vi "Std_dilution_SubVI_BM.vi"(6 "COM Port":refnum<visa-resource-name>="COM9", 7 "Pump Parameters":T1={"Speed 1"="100", "Speed 2"="250", "Speed 3"="250", "Speed 4"="250", "UW/Sample"="5", "Sparge"="2", "Std"="4", "Waste"="15", "Air"="14", "Milli-Q"="1", "H2SO4"="6", "NaOH"="3", "Catalyst"="7", "Cell (H+ side)"="8", "Cell (sample side)"="9", "NaCl"="9"}, 9 "step to ml":dbl=1920.0, 10 "Total Vol. (mL)":dbl, 11 "Dilution Vol. (mL)":dbl=10.0) -> ()   [LabVIEW 2021]
panel:
  out "Full Command":string="o4A0V5000o1P14400o4D14400o1P33600o4D9600o2D24000o5P9600o2D9600o6P33600o4D33600"
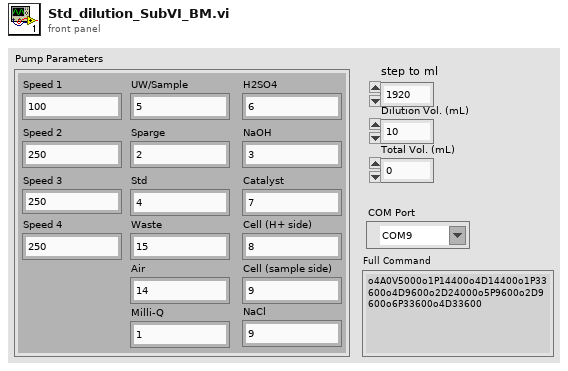
[diagram p1: front panel]
types:
  T1 = cluster{"Speed 1":string, "Speed 2":string, "Speed 3":string, "Speed 4":string, "UW/Sample":string, "Sparge":string, "Std":string, "Waste":string, "Air":string, "Milli-Q":string, "H2SO4":string, "NaOH":string, "Catalyst":string, "Cell (H+ side)":string, "Cell (sample side)":string, "NaCl":string}
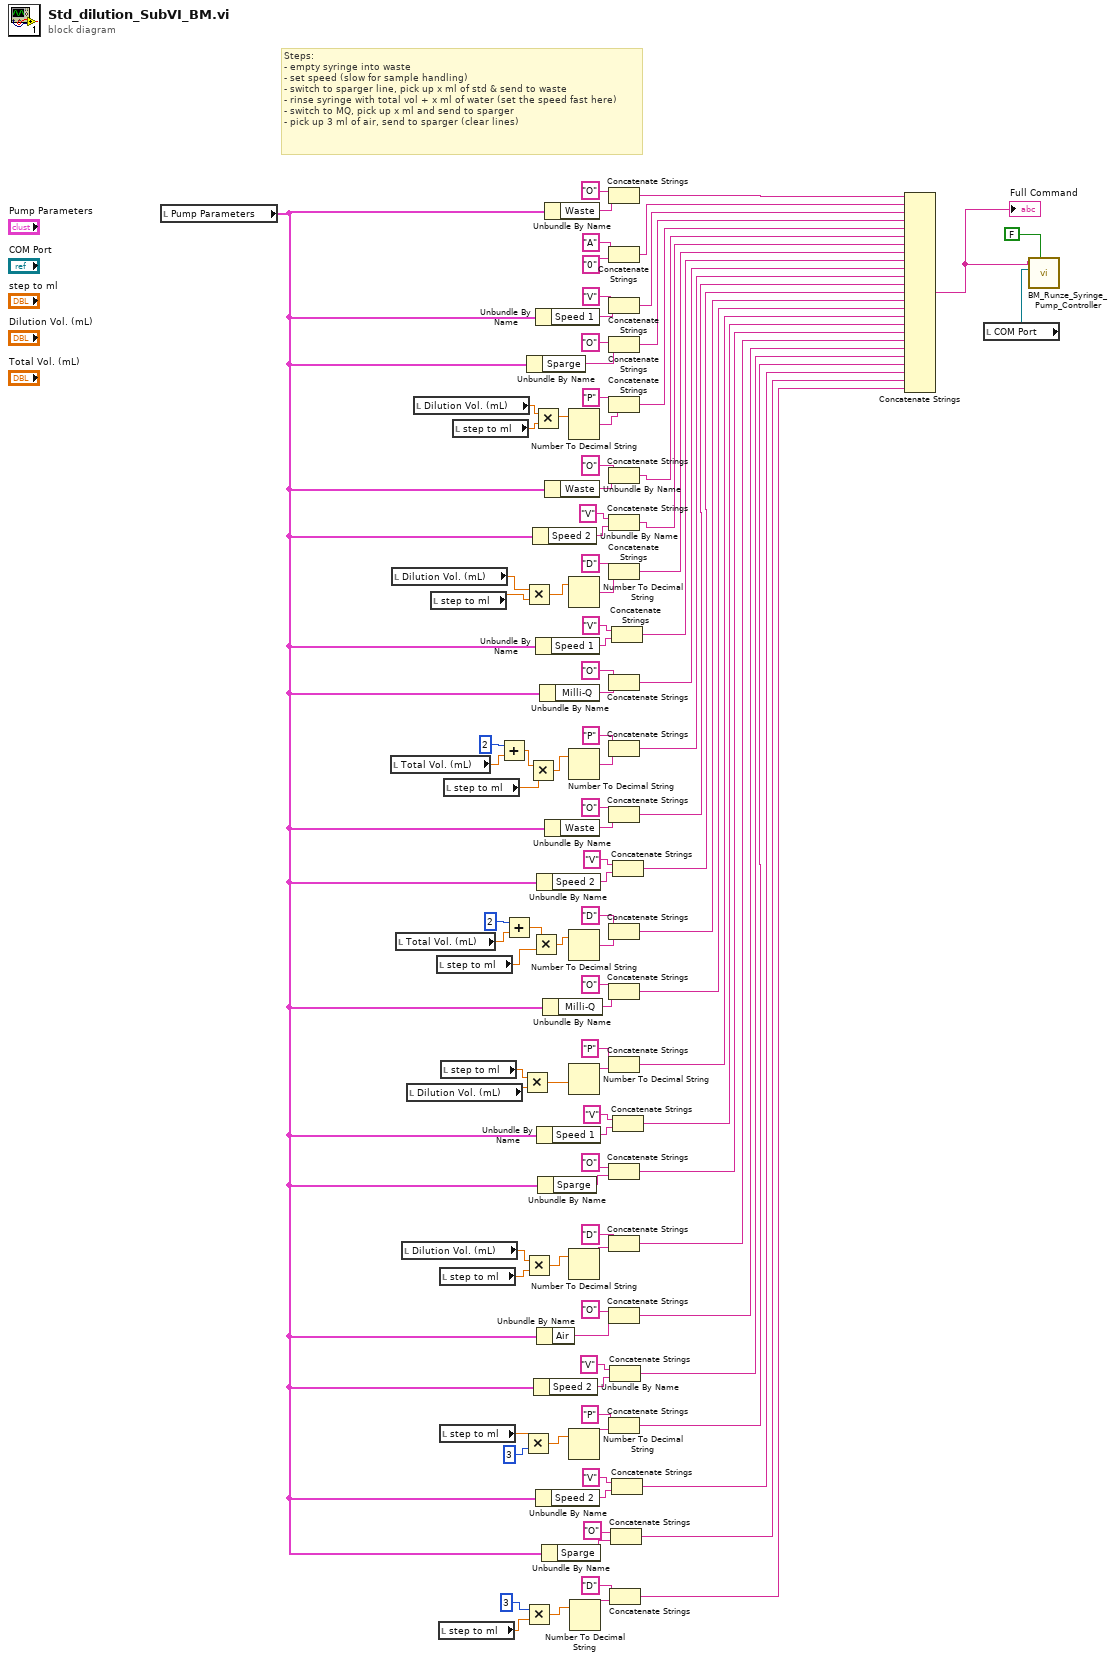
[diagram p0: block diagram]
diagram:
  # "Steps:\n- empty syringe into waste\n- set speed (slow for sample handling)\n- switch to sparger line, pick up x ml of std & send to waste\n- rinse syringe with total vol + x ml of water (set the speed fast here)\n- switch to MQ, pick up x ml and send to sparger\n- pick up 3 ml of air, send to sparger (clear lines)"
  n1 = local read "Pump Parameters"() -> (w10:T1)
  n2 = local read "Total Vol. (mL)"() -> (w77:dbl)
  n3 = local read "Dilution Vol. (mL)"() -> (w8:dbl)
  n4 = local read "Total Vol. (mL)"() -> (w7:dbl)
  n5 = local read "Dilution Vol. (mL)"() -> (w3:dbl)
  n6 = local read "Dilution Vol. (mL)"() -> (w76:dbl)
  n7 = local read "Dilution Vol. (mL)"() -> (w9:dbl)
  n8 = local read "step to ml"() -> (w72:dbl)
  n9 = local read "step to ml"() -> (w5:dbl)
  n10 = local read "step to ml"() -> (w13:dbl)
  n11 = local read "step to ml"() -> (w2:dbl)
  n12 = local read "step to ml"() -> (w61:dbl)
  n13 = local read "step to ml"() -> (w87:dbl)
  n14 = local read "step to ml"() -> (w88:dbl)
  n15 = local read "step to ml"() -> (w89:dbl)
  n16 = Add(x=2, y=w77) -> (x+y=w102:dbl)
  n17 = Add(x=2, y=w7) -> (x+y=w4:dbl)
  n18 = Multiply(x=w87, y=w76) -> (x*y=w105:dbl)
  n19 = Multiply(x=w61, y=3) -> (x*y=w62:dbl)
  n20 = Multiply(x=w8, y=w72) -> (x*y=w73:dbl)
  n21 = Multiply(x=w3, y=w2) -> (x*y=w104:dbl)
  n22 = Multiply(x=3, y=w13) -> (x*y=w16:dbl)
  n23 = Unbundle By Name(w10) -> ("Sparge"=w84:string)
  n24 = Multiply(x=w102, y=w88) -> (x*y=w103:dbl)
  n25 = Multiply(x=w4, y=w5) -> (x*y=w106:dbl)
  n26 = Multiply(x=w9, y=w89) -> (x*y=w101:dbl)
  n27 = Unbundle By Name(w10) -> ("Speed 2"=w54:string)
  n28 = Unbundle By Name(w10) -> ("Speed 2"=w46:string)
  n29 = Unbundle By Name(w10) -> ("Speed 1"=w85:string)
  n30 = Unbundle By Name(w10) -> ("Speed 1"=w53:string)
  n31 = Unbundle By Name(w10) -> ("Speed 2"=w45:string)
  n32 = Unbundle By Name(w10) -> ("Speed 2"=w50:string)
  n33 = Unbundle By Name(w10) -> ("Speed 1"=w49:string)
  n34 = Unbundle By Name(w10) -> ("Air"=w78:string)
  n35 = Unbundle By Name(w10) -> ("Sparge"=w79:string)
  n36 = Unbundle By Name(w10) -> ("Milli-Q"=w82:string)
  n37 = Unbundle By Name(w10) -> ("Sparge"=w17:string)
  n38 = Unbundle By Name(w10) -> ("Milli-Q"=w80:string)
  n39 = Unbundle By Name(w10) -> ("Waste"=w86:string)
  n40 = Unbundle By Name(w10) -> ("Waste"=w83:string)
  n41 = Unbundle By Name(w10) -> ("Waste"=w81:string)
  n42 = Number To Decimal String(number=w101) -> (decimal integer string=w71:string)  [unwired: 1 out]
  n43 = Number To Decimal String(number=w73) -> (decimal integer string=w70:string)  [unwired: 1 out]
  n44 = Number To Decimal String(number=w103) -> (decimal integer string=w68:string)  [unwired: 1 out]
  n45 = Number To Decimal String(number=w106) -> (decimal integer string=w67:string)  [unwired: 1 out]
  n46 = Number To Decimal String(number=w105) -> (decimal integer string=w64:string)  [unwired: 1 out]
  n47 = Number To Decimal String(number=w104) -> (decimal integer string=w59:string)  [unwired: 1 out]
  n48 = Number To Decimal String(number=w62) -> (decimal integer string=w57:string)  [unwired: 1 out]
  n49 = Number To Decimal String(number=w16) -> (decimal integer string=w14:string)  [unwired: 1 out]
  n50 = Concatenate Strings("O", w86) -> (w42:string)
  n51 = Concatenate Strings("A", "0") -> (w41:string)
  n52 = Concatenate Strings("V", w85) -> (w40:string)
  n53 = Concatenate Strings("O", w84) -> (w39:string)
  n54 = Concatenate Strings("P", w71) -> (w38:string)
  n55 = Concatenate Strings("O", w83) -> (w37:string)
  n56 = Concatenate Strings("V", w54) -> (w36:string)
  n57 = Concatenate Strings("D", w70) -> (w35:string)
  n58 = Concatenate Strings("O", w82) -> (w33:string)
  n59 = Concatenate Strings("P", w68) -> (w32:string)
  n60 = Concatenate Strings("O", w81) -> (w31:string)
  n61 = Concatenate Strings("D", w67) -> (w29:string)
  n62 = Concatenate Strings("O", w80) -> (w28:string)
  n63 = Concatenate Strings("P", w64) -> (w27:string)
  n64 = Concatenate Strings("O", w79) -> (w25:string)
  n65 = Concatenate Strings("D", w59) -> (w24:string)
  n66 = Concatenate Strings("O", w78) -> (w23:string)
  n67 = Concatenate Strings("P", w57) -> (w21:string)
  n68 = Concatenate Strings("V", w46) -> (w22:string)
  n69 = Concatenate Strings("D", w14) -> (w11:string)
  n70 = Concatenate Strings("O", w17) -> (w12:string)
  n71 = Concatenate Strings("V", w53) -> (w34:string)
  n72 = Concatenate Strings("V", w45) -> (w20:string)
  n73 = Concatenate Strings("V", w50) -> (w30:string)
  n74 = Concatenate Strings("V", w49) -> (w26:string)
  n75 = Concatenate Strings(w42, w41, w40, w39, w38, w37, w36, w35, w34, w33, w32, w31, w30, w29, w28, w27, w26, w25, w24, w23, w22, w21, w20, w12, w11) -> (w92:string)
  "Full Command" <- w92
  n76 = local read "COM Port"() -> (w91:refnum<visa-resource-name>)
  n77 = call "BM_Runze_Syringe_Pump_Controller.vi"("Initialize Plunger?"=FALSE ("Initialize?"), "COM Port (Runze)"=w91, "Enter Command"=w92) -> ()  [unwired: 6 in, 3 out]
